vi "WLAN_ChannelEstimation.vi"(11 "LTF":cdb[](array[numeric])) -> (3 "Frequency estimation":cdb[](array[numeric]))   [LabVIEW 2014]
uses:
  <vilib>/Analysis/2dsp.llb/Complex FFT.vi
  <vilib>/Analysis/NI_AALPro.lvlib
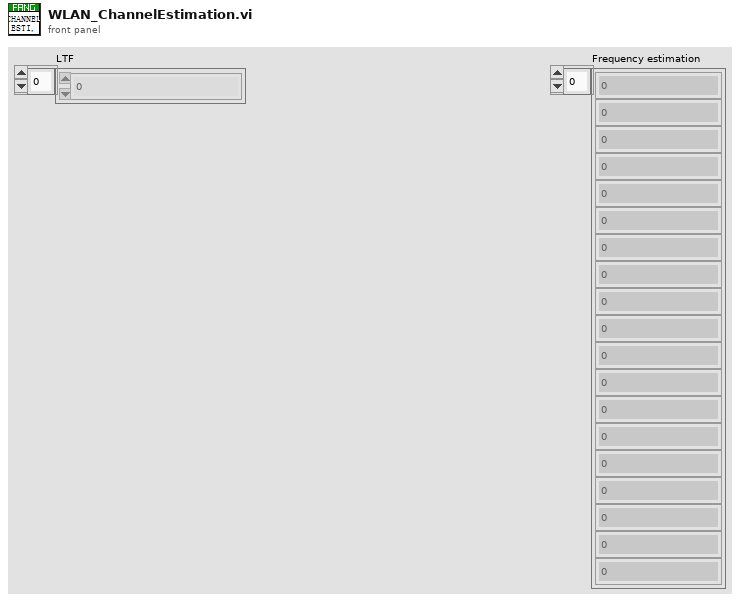
[diagram p1: front panel]
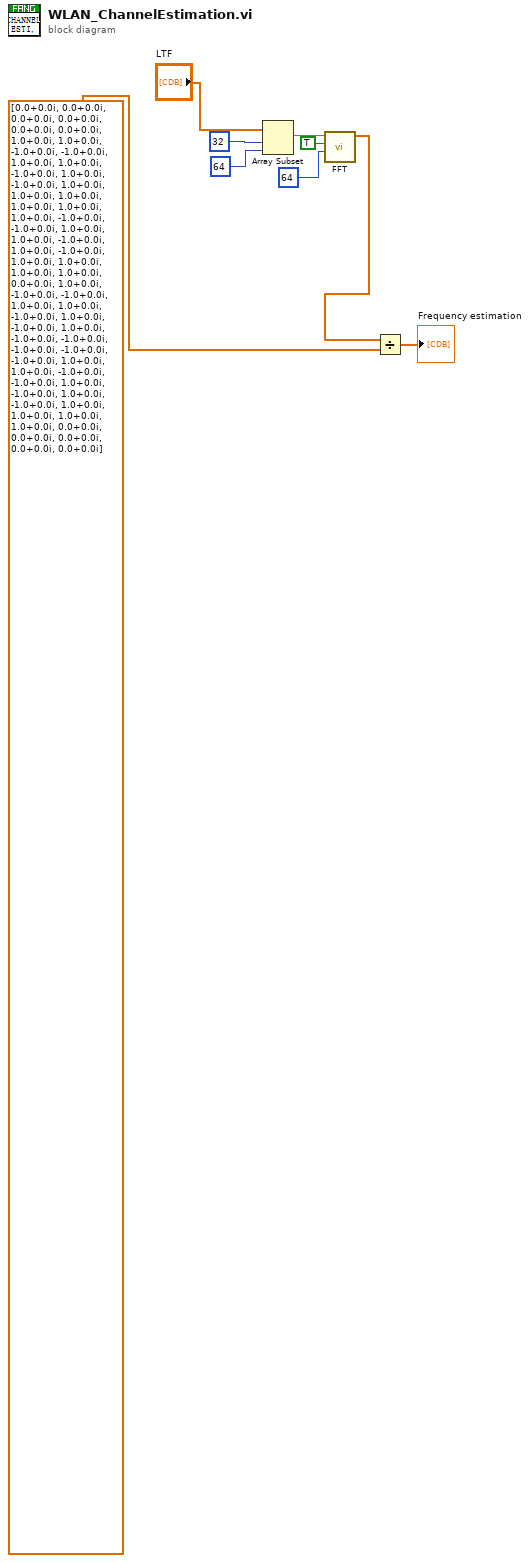
[diagram p0: block diagram]
diagram:
  n1 = Array Subset(array="LTF", index=32, length=64) -> (w5:cdb[])
  n2 = call-poly <vilib>:"FFT.vi"("FFT size"=64, "shift?"=TRUE, "X"=w5) -> ("FFT {X}"=w2:cdb[])  [unwired: 7 in, 1 out]
  n3 = Divide(x=w2, y=cdb[] [0.0+0.0i, 0.0+0.0i, 0.0+0.0i, 0.0+0.0i, 0.0+0.0i, 0.0+0.0i, 1.0+0.0i, 1.0+0.0i, -1.0+0.0i, -1.0+0.0i, 1.0+0.0i, 1.0+0.0i, -1.0+0.0i, 1.0+0.0i, -1.0+0.0i, 1.0+0.0i, 1.0+0.0i, 1.0+0.0i, 1.0+0.0i, 1.0+0.0i, 1.0+0.0i, -1.0+0.0i, -1.0+0.0i, 1.0+0.0i, 1.0+0.0i, -1.0+0.0i, 1.0+0.0i, -1.0+0.0i, 1.0+0.0i, 1.0+0.0i, 1.0+0.0i, 1.0+0.0i, 0.0+0.0i, 1.0+0.0i, -1.0+0.0i, -1.0+0.0i, 1.0+0.0i, 1.0+0.0i, -1.0+0.0i, 1.0+0.0i, -1.0+0.0i, 1.0+0.0i, -1.0+0.0i, -1.0+0.0i, -1.0+0.0i, -1.0+0.0i, -1.0+0.0i, 1.0+0.0i, 1.0+0.0i, -1.0+0.0i, -1.0+0.0i, 1.0+0.0i, -1.0+0.0i, 1.0+0.0i, -1.0+0.0i, 1.0+0.0i, 1.0+0.0i, 1.0+0.0i, 1.0+0.0i, 0.0+0.0i, 0.0+0.0i, 0.0+0.0i, 0.0+0.0i, 0.0+0.0i]) -> (x/y=→"Frequency estimation":cdb[])
